vi "Write Request Headers.vi"(8 "error in (no error)":errorcluster, 10 "Request Headers":T1[](array[typedef]), 11 "REST Interface in":refnum<class "REST Interface.lvclass">) -> (0 "error out":errorcluster, 3 "REST Interface out":refnum<class "REST Interface.lvclass">)   [LabVIEW 2018, in "REST Interface.lvlib" / "REST Interface.lvclass"]
uses:
  REST Interface.lvclass
  <vilib>/addons/_JKI.lib/REST Client/classes/REST Client/HTTP Header.ctl
  REST Interface.lvclass/REST Interface.ctl
  <vilib>/addons/_JKI.lib/REST Client/classes/REST Client/REST Client.lvclass
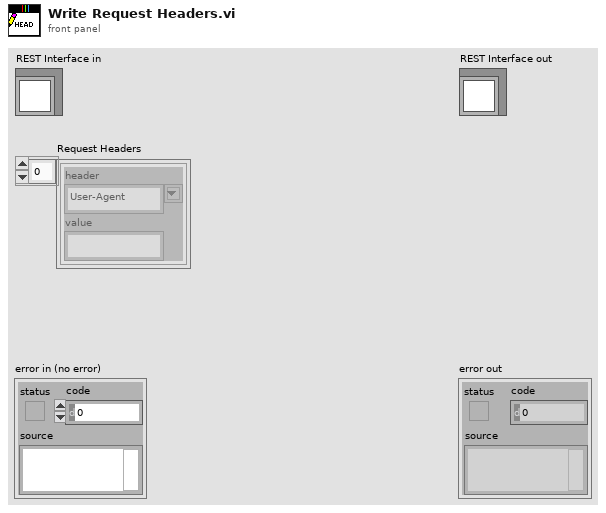
[diagram p1: front panel]
types:
  T1 = typedef "REST Client.lvlib/REST Client.lvclass/HTTP Header.ctl" = cluster{"header":string, "value":string}
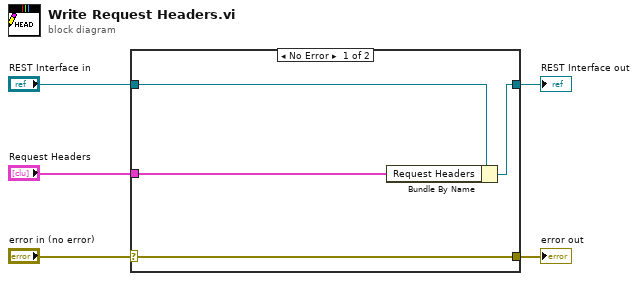
[diagram p0: block diagram]
diagram:
  n1 = case shown="No Error" "error in (no error)" {
    selector: "error in (no error)" -> [w9 w10]
    tunnel: [w9 w10] -> w4
    tunnel: [w7 w11] -> w2
    tunnel: "REST Interface in" -> [w8 w11]
    tunnel: "Request Headers" -> [w6 _]
    frame No Error {
      n2 = Bundle By Name(cluster=w8, "Request Headers"=w6) -> (w7:refnum<class "REST Interface.lvclass">)
    }
    frame Error {
    }
  }
  "error out" <- w4
  "REST Interface out" <- w2
